vi "Vision Processing.vi"(4 "error in (no error)":errorcluster, 5 "Test":bool, 7 "Image Size":T1=enum."Custom") -> ()   [LabVIEW 2016]
doc: "This VI runs in parallel to other tasks. It gets images from the camera, processes them for color or shape and use that information to affect robot behavior."
uses:
  <vilib>/Rock Robotics/WPI/Camera/WPI_CameraImageSize.ctl
  <vilib>/Rock Robotics/WPI/Camera/WPI_CameraWhite Balance Values.ctl
  <vilib>/Rock Robotics/WPI/Camera/WPI_CameraExposure Values.ctl
  <vilib>/Rock Robotics/WPI/Camera/WPI_CameraFrameRate.ctl
  Robot Global Data.vi
  Global 4.vi
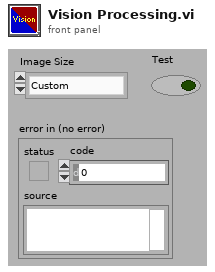
[diagram p1: front panel]
types:
  T1 = typedef "WPI_CameraImageSize.ctl" = enum16{"640x480", "320x240", "160x120", "Custom"}
  T2 = typedef "WPI_CameraFrameRate.ctl" = u32
  T3 = typedef "WPI_CameraExposure Values.ctl" = enum16{"Auto", "Flicker-free 50 Hz", "Flicker-free 60 Hz", "Hold current", "Custom"}
  T4 = typedef "WPI_CameraWhite Balance Values.ctl" = enum16{"Auto", "Fixed indoor", "Fixed outdoor 1", "Fixed outdoor 2", "Fixed fluorescent 1", "Fixed fluorescent 2", "Hold current", "Custom"}
  T5 = typedef "Image Type" = u32
  T6 = typedef "WPI_CameraDevRef.ctl" = cluster{"Camera Address":string, "CameraStatus":errorcluster}
  T7 = typedef "IMAQ Image.ctl" = refnum<image>
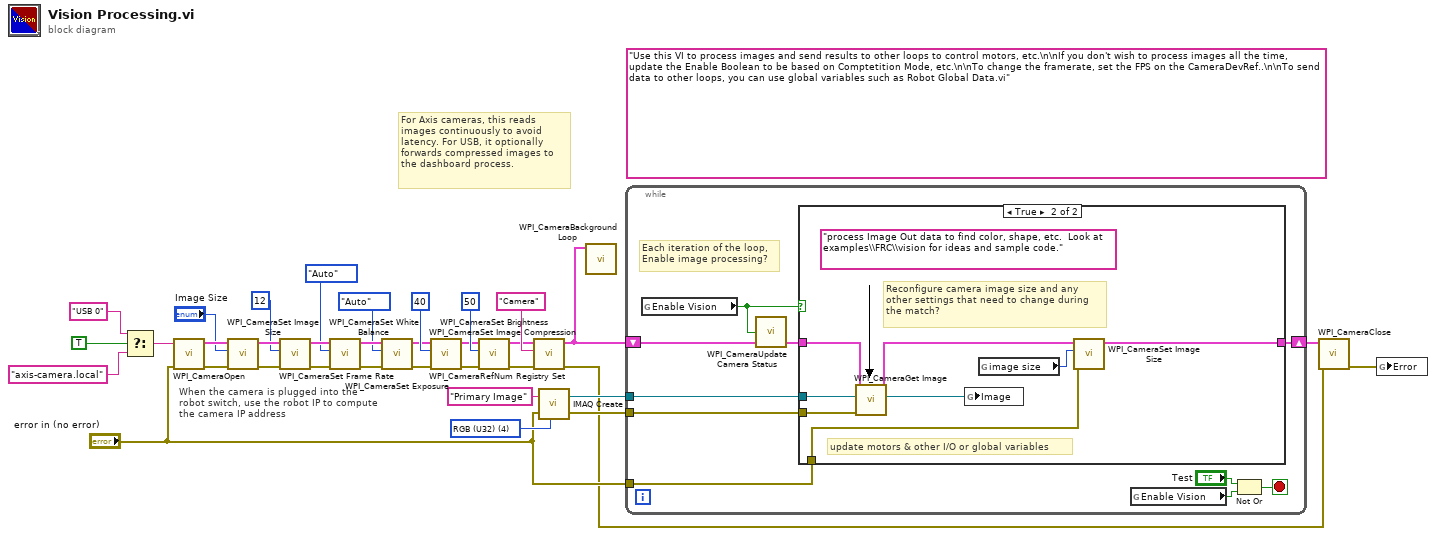
[diagram p0: block diagram]
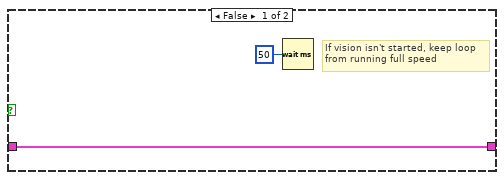
[diagram p2: hidden frame]
diagram:
  (unwired) "Use this VI to process images and send results to other loops to control motors, etc.\n\nIf you don't wish to process images all the time, update the Enable Boolean to be based on Comptetition Mode, etc.\n\nTo change the framerate, set the FPS on the CameraDevRef..\n\nTo send data to other loops, you can use global variables such as Robot Global Data.vi"
  w34 = T5 4 items=["Grayscale (U8)", "Grayscale (I16)", "Grayscale (SGL)", "Complex (CSG)", "RGB (U32)", "HSL (U32)", "RGB (U64)"] ("Image Type")
  # "When the camera is plugged into the\nrobot switch, use the robot IP to compute\nthe camera IP address"
  # "For Axis cameras, this reads\nimages continuously to avoid\nlatency. For USB, it optionally\nforwards compressed images to\nthe dashboard process."
  n1 = Select(t="USB 0" ("format string"), s=TRUE ("dot notation? (F)"), f="axis-camera.local" ("format string")) -> (s? t:f=w6:string)
  n2 = call <vilib>:"WPI_CameraOpen.vi"("error in (no error)"="error in (no error)", "Camera Address"=w6) -> ("error out"=w22:errorcluster, "CameraDevRef"=w23:T6)  [unwired: 1 in, 7 out]
  n3 = call <vilib>:"WPI_CameraSet Image Size.vi"("error in (no error)"=w22, "Image Size"="Image Size", "CameraDevRef"=w23) -> ("error out"=w21:errorcluster, "CameraDevRef Out"=w24:T6)  [unwired: 1 in, 6 out]
  n4 = call <vilib>:"WPI_CameraSet Frame Rate.vi"("error in (no error)"=w21, "Frame Rate (fps)"=T2 12, "CameraDevRef"=w24) -> ("error out"=w20:errorcluster, "CameraDevRef Out"=w26:T6)  [unwired: 7 out]
  n5 = call <vilib>:"WPI_CameraSet White Balance.vi"("error in (no error)"=w20, "White Balance"=WPI_CameraWhite_Balance_Values."Auto", "CameraDevRef"=w26) -> ("error out"=w19:errorcluster, "CameraDevRef Out"=w25:T6)  [unwired: 1 in, 6 out]
  n6 = call <vilib>:"WPI_CameraSet Exposure.vi"("error in (no error)"=w19, "Exposure"=WPI_CameraExposure_Values."Auto", "CameraDevRef"=w25) -> ("error out"=w18:errorcluster, "CameraDevRef Out"=w28:T6)  [unwired: 1 in, 6 out]
  n7 = call <vilib>:"WPI_CameraSet Image Compression.vi"("error in (no error)"=w18, "Compression"=40, "CameraDevRef"=w28) -> ("error out"=w17:errorcluster, "CameraDevRef Out"=w27:T6)  [unwired: 7 out]
  n8 = call <vilib>:"WPI_CameraSet Brightness.vi"("error in (no error)"=w17, "Brightness"=50, "CameraDevRef"=w27) -> ("error out"=w15:errorcluster, "CameraDevRef Out"=w16:T6)  [unwired: 7 out]
  n9 = call <vilib>:"WPI_CameraRefNum Registry Set.vi"("error in (no error)"=w15, "refnum name"="Camera", "CameraDevRef"=w16) -> ("error out"=w2:errorcluster, "CameraDevRef"=w11:T6)  [unwired: 1 in, 6 out]
  n10 = call "IMAQ Create"("Image Name"="Primary Image", "Image Type"=w34, "error in (no error)"="error in (no error)") -> ("New Image"=w32:T7, "error out"=w4:errorcluster)  [unwired: 1 in, 1 out]
  n11 = call <vilib>:"WPI_CameraBackground Loop.vi"("CameraDevRef"=w11) -> ()  [unwired: 11 in]
  n12 = while {
    shift-right: [w44] -> w9
    shift-left: w11 -> [w42]
    tunnel: w32 -> [w43]
    tunnel: "error in (no error)" -> [w39]
    tunnel: w4 -> [w38]
    stop <- w37 stop-if-true
    # "Each iteration of the loop,\nEnable image processing?"
    n13 = global read "Robot Global Data.vi" "Enable Vision"() -> (w40:bool)
    n14 = call <vilib>:"WPI_CameraUpdate Camera Status.vi"("CameraDevRef In"=w42, "Enable Vision"=w40) -> ("CameraDevRef Out"=w41:T6)  [unwired: 3 in]
    n15 = case shown="True" w40 {
      tunnel: w43 -> [_ w53]
      tunnel: [w46 w54] -> w44
      tunnel: w41 -> [w46 w52]
      tunnel: w39 -> [_ w50]
      tunnel: w38 -> [_ w49]
      frame False {
        # "If vision isn't started, keep loop\nfrom running full speed"
        n16 = Wait (ms)(milliseconds to wait=u32 50) -> ()  [unwired: 1 out]
      }
      frame True {
        (unwired) "process Image Out data to find color, shape, etc.  Look at examples\\FRC\\vision for ideas and sample code."
        # "update motors & other I/O or global variables"
        # "Reconfigure camera image size and any\nother settings that need to change during\nthe match?"
        n17 = call <vilib>:"WPI_CameraGet Image.vi"("error in (no error)"=w49, "Image"=w53, "CameraDevRef"=w52) -> ("Image Out"=w47:T7, "CameraDevRef Out"=w51:T6)  [unwired: 7 out]
        n18 = global write "Global 4.vi" "Image"(w47) -> ()
        n19 = global read "Robot Global Data.vi" "image size"() -> (w48:T1)
        n20 = call <vilib>:"WPI_CameraSet Image Size.vi"("error in (no error)"=w50, "Image Size"=w48, "CameraDevRef"=w51) -> ("CameraDevRef Out"=w54:T6)  [unwired: 1 in, 7 out]
      }
    }
    n21 = global read "Robot Global Data.vi" "Enable Vision"() -> (w35:bool)
    n22 = Not Or(1:w35, 2:"Test") -> (0:w37:bool)
  }
  n23 = call <vilib>:"WPI_CameraClose.vi"("error in (no error)"=w2, "CameraDevRef"=w9) -> ("error out"=w1:errorcluster)  [unwired: 9 out]
  n24 = global write "Global 4.vi" "Error"(w1) -> ()
